vi "CSM Data Type String to Enum(TypeEnum).vi"(10 "Data Type String":string) -> (1 "Array Dim":i32, 2 "Secondary Type":T1, 3 "Primary Type":T1)   [LabVIEW 2017, in "Communicable State Machine.lvlib"]
doc: "Converts a data type description string into a LabVIEW-defined data type enum and returns the array subtype using an enum.\n\n-- <b>Controls</b> --\n- <b>Data Type String</b>: Input data type description string.\n\n-- <b>Indicators</b> --\n- <b>Primary Type</b>: Data type enum.\n- <b>Secondary Type String</b>: Array subtype enum.\n- <b>Array Dim</b>: If the input is an array data type, returns the array dimensions."
uses:
  Communicable State Machine.lvlib
  <vilib>/Utility/Data Type/Type Definitions/Data Type.ctl
  <vilib>/Utility/Data Type/NI_Data Type.lvlib
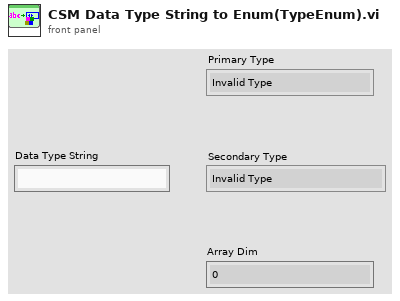
[diagram p1: front panel]
types:
  T1 = typedef "NI_Data Type.lvlib/Data Type.ctl" = enum8{"Invalid Type", "Void", "I8", "I16", "I32", "I64", "U8", "U16", "U32", "U64", "Single Float", "Double Float", "Extended Float", "Single Complex", "Double Complex", "Extended Complex", "Enum U8", "Enum U16", "Enum U32", "Enum U64", "Single Float With Unit", "Double Float With Unit", "Extended Float With Unit", "Single Complex with Unit", "Double Complex with Unit", "Extended Complex with Unit", "Boolean", "String", "Path", "Picture", "Tag", "Array", "Cluster", "Variant", "LV Variant", "Waveform", "Timestamp", "Digital Waveform", "Digital Data", "ExpressData", "Refnum", "External Data", "VI", "Poly VI", "LabVIEW Class Instance", "Fixed Point"}
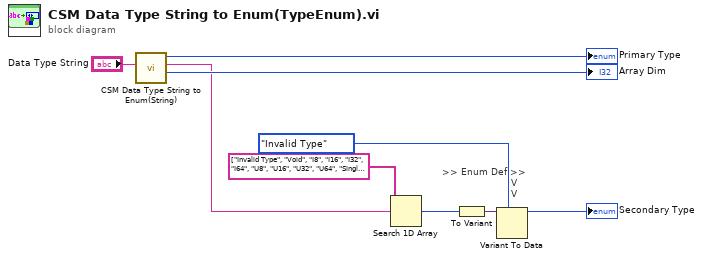
[diagram p0: block diagram]
diagram:
  # ">> Enum Def >>\n                       V\n                       V"
  n1 = call "CSM Data Type String to Enum(String).vi"("Data Type String"="Data Type String") -> ("Array Dim"=→"Array Dim":i32, "Secondary Type String"=w2:string, "Primary Type"=→"Primary Type":T1)  [unwired: 8 in]
  n2 = Search 1D Array(1D array=string[] ["Invalid Type", "Void", "I8", "I16", "I32", "I64", "U8", "U16", "U32", "U64", "Single Float", "Double Float", "Extended Float", "Single Complex", "Double Complex", "Extended Complex", "Enum U8", "Enum U16", "Enum U32", "Enum U64", "Single Float With Unit", "Double Float With Unit", "Extended Float With Unit", "Single Complex with Unit", "Double Complex with Unit", "Extended Complex with Unit", "Boolean", "String", "Path", "Picture", "Tag", "Array", "Cluster", "Variant", "LV Variant", "Waveform", "Timestamp", "Digital Waveform", "Digital Data", "ExpressData", "Refnum", "External Data", "VI", "Poly VI", "LabVIEW Class Instance", "Fixed Point"] ("Enum Strings"), element=w2) -> (index of element=w4:i32)  [unwired: 1 in]
  n3 = To Variant(anything=w4) -> (Variant=w6:variant)
  n4 = Variant To Data(type=Data_Type."Invalid Type" ("Type"), Variant=w6) -> (data=→"Secondary Type":T1)  [unwired: 1 in, 1 out]
